vi "Untitled 3 emibin log11.vi"() -> ()   [LabVIEW 2011]
uses:
  Host Code/emi cndiates/bin File/Log emibin/Log11/Ch Info dbl.ctl
  Host Code/emi cndiates/bin File/Log emibin/Log11/Ch Info u8 std.ctl
  Host Code/emi cndiates/bin File/Log emibin/Log11/Log11 emibin file Metrix.ctl
panel:
  in  "File type ID(0, generic)":u16
  in  "File type Version(0, Unset)":u8
  in  "File sub type(All)":u16=65535
  in  "File sub type":u8=1
  out "Log11 File Metrix":T1
  out "Write time":u32
  out "Result":cluster{"current time":timestamp, dbl[], u8[]}[](array[cluster])
  out "dbl Array result":T2[](array[typedef])
  out "u8 std Array result":T3[](array[typedef])
  out "Read time":u32
  in  "u8 std Array":T3[](array[typedef])
  in  "dbl Array":T2[](array[typedef])
  in  "Numb data sets":i32
  out "Corrupt":bool
  out "error out":errorcluster
  out "Sets of data":u32
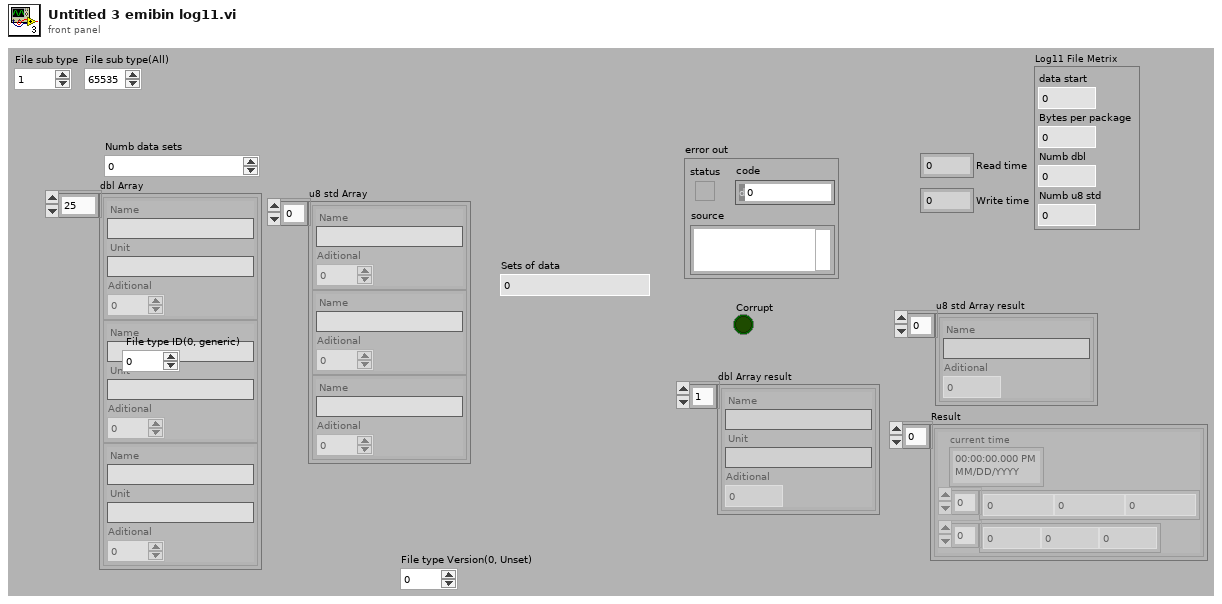
[diagram p1: front panel]
types:
  T1 = typedef "Log11 emibin file Metrix.ctl" = cluster{"data start":u32, "Bytes per package":i32, "Numb dbl":i32, "Numb u8 std":i32}
  T2 = typedef "Ch Info dbl.ctl" = cluster{"Name":string, "Unit":string, "Aditional":i32}
  T3 = typedef "Ch Info u8 std.ctl" = cluster{"Name":string, "Aditional":i32}
  T4 = cluster{"record time":timestamp, "Doubles":dbl[], "U8 std":u8[]}
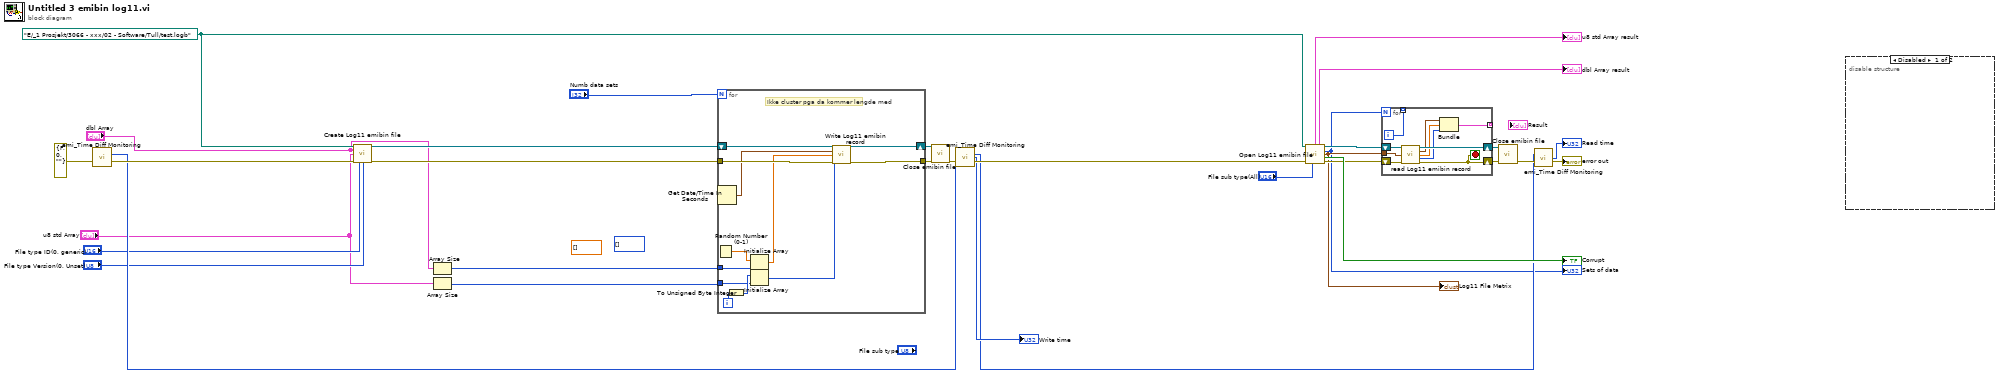
[diagram p0: block diagram]
diagram:
  (unwired) u8[] [] ("initialized array")
  (unwired) dbl[] [] ("initialized array")
  w32 = path "E:/_1 Prosjekt/3066 - xxx/02 - Software/Tull/test.logb" ("file path")
  n1 = call "emi_Time Diff Monitoring.vi"("error in (no error)"=errorcluster {"status"=FALSE, "code"=0, "source"=""}) -> ("Current Time"=w13:u32, "error out"=w21:errorcluster)  [unwired: 12 in, 1 out]
  n2 = call "Create Log11 emibin file.vi"("file path"=w32, "dbl Array"="dbl Array", "u8 std Array"="u8 std Array", "error in"=w21, "File type ID(0, generic)"="File type ID(0, generic)", "File type Version(0, Unset)"="File type Version(0, Unset)") -> ("refnum out"=w27:refnum<file>, "error out"=w29:errorcluster)  [unwired: 8 in]
  n3 = Array Size(array="dbl Array") -> (size(s)=w25:i32)
  n4 = Array Size(array="u8 std Array") -> (size(s)=w24:i32)
  n5 = for {
    N: "Numb data sets" -> [_]
    tunnel: w29 -> [w39]
    tunnel: [w37] -> w28
    tunnel: w25 -> [w43]
    tunnel: w24 -> [w40]
    shift-right: [w36] -> w26
    shift-left: w27 -> [w38]
    i -> [w41]
    # "Ikke cluster pga da kommer lengde med"
    n6 = Random Number (0-1)() -> (number: 0 to 1=w44:dbl)
    n7 = Get Date/Time In Seconds() -> (seconds since 1Jan1904=w35:timestamp)
    n8 = To Unsigned Byte Integer(number=w41) -> (unsigned 8bit integer=w42:u8)
    n9 = Initialize Array(w44, w43) -> (w34:dbl[])
    n10 = Initialize Array(w42, w40) -> (w33:u8[])
    n11 = call "Write Log11 emibin record.vi"("refnum in"=w38, "Time"=w35, "Doubles"=w34, "u8"=w33, "error in"=w39) -> ("refnum out"=w36:refnum<file>, "error out"=w37:errorcluster)  [unwired: 9 in]
  }
  n12 = call "Close emibin file.vi"("refnum in"=w26, "error in (no error)"=w28) -> ("error out"=w16:errorcluster)  [unwired: 13 in]
  n13 = call "emi_Time Diff Monitoring.vi"("Previous Time"=w13, "error in (no error)"=w16) -> ("Current Time"=w12:u32, "Time Difference(ms)"=→"Write time":u32, "error out"=w15:errorcluster)  [unwired: 11 in]
  n14 = call "Open Log11 emibin file.vi"("file path"=w32, "error in"=w15, "File sub type(All)"="File sub type(All)") -> ("u8 std Array"=→"u8 std Array result":T3[], "dbl Array"=→"dbl Array result":T2[], "refnum out"=w10:refnum<file>, "Numb packages"=w8:i64, "Log11 File Metrix"=w9:T1, "Corrupt"=→"Corrupt":bool, "error out"=w11:errorcluster)  [unwired: 6 in]
  "Sets of data" <- w8
  "Log11 File Metrix" <- w9
  n15 = for {
    N: w8 -> [_]
    shift-right: [w46] -> w7
    shift-left: w11 -> [w54]
    shift-right: [w52] -> w6
    shift-left: w10 -> [w53]
    tunnel: w9 -> [w47]
    tunnel: [w48] -> _ mode=indexing
    tunnel: [w45] -> _ mode=indexing
    i -> [w45]
    stop <- w46 stop-if-true
    n16 = call "read Log11 emibin record.vi"("refnum in"=w53, "Log11 File Metrix"=w47, "error in"=w54) -> ("refnum out"=w52:refnum<file>, "record time"=w51:timestamp, "Doubles"=w50:dbl[], "U8 std"=w49:u8[], "error out"=w46:errorcluster)  [unwired: 8 in]
    n17 = Bundle("record time"=w51, "Doubles"=w50, "U8 std"=w49) -> (w48:T4)  [unwired: 1 in]
  }
  n18 = call "Close emibin file.vi"("refnum in"=w6, "error in (no error)"=w7) -> ("error out"=w31:errorcluster)  [unwired: 13 in]
  n19 = call "emi_Time Diff Monitoring.vi"("Previous Time"=w12, "error in (no error)"=w31) -> ("Time Difference(ms)"=→"Read time":u32, "error out"=→"error out":errorcluster)  [unwired: 11 in, 1 out]
  n20 = disable-structure shown="Disabled" {
    frame Disabled {
    }
    frame Enabled {
    }
  }
